vi "messageToCommand.vi"(7 "Self Enqueuer":refnum<class "Message Enqueuer.lvclass">, 8 "error in (no error)":errorcluster, 10 "Arguments":variant, 11 "Command":string) -> (0 "error out":errorcluster)   [LabVIEW 2017, in "BuildWorker.lvlib" / "BuildWorker.lvclass"]
uses:
  BuildWorker.lvclass
  <vilib>/ActorFramework/Message Enqueuer/Message Enqueuer.lvclass
  <vilib>/ActorFramework/Message Enqueuer/Message Enqueuer.lvclass/Message Enqueuer.ctl
  <vilib>/ActorFramework/Message Enqueuer/Enqueue.vi
  <vilib>/ActorFramework/Stop Msg/Stop Msg.lvclass
  Applications/National Instruments/LabVIEW 2017 64-bit/vi.lib/ActorFramework/Message/Message.lvclass
  WebSocket Server/Actors/Actor wHelper/Actor wUI Messages/Show UI Msg/Show UI Msg.lvclass
  <vilib>/ActorFramework/Message Priority Queue/Priority Enqueue.vi
  BuildWorker Messages/Name Request Msg/Name Request Msg.lvclass
  BuildWorker Messages/Remove Task Request Msg/Remove Task Request Msg.lvclass
  BuildWorker Messages/CurrentTaskName Request Msg/CurrentTaskName Request Msg.lvclass
  BuildWorker Messages/New Task Request Msg/New Task Request Msg.lvclass
  BuildWorker Messages/Enqueue Task List Msg/Enqueue Task List Msg.lvclass
  BuildWorker Messages/Abort Msg/Abort Msg.lvclass
  BuildWorker Messages/Send Worker Status Update Msg/Send Worker Status Update Msg.lvclass
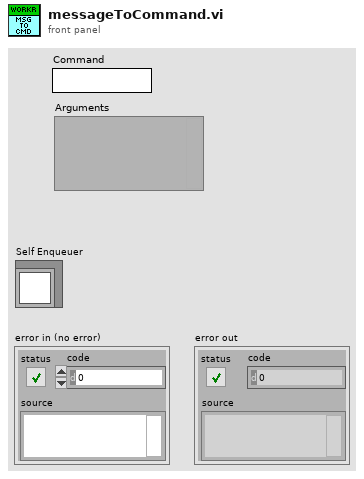
[diagram p1: front panel]
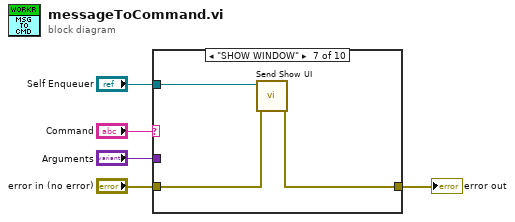
[diagram p0: block diagram]
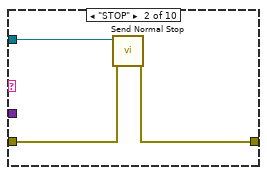
[diagram p3: hidden frame]
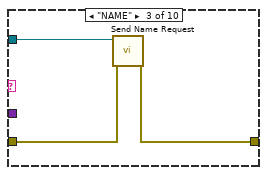
[diagram p4: hidden frame]
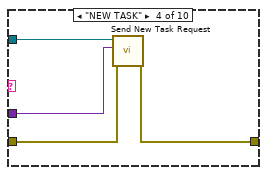
[diagram p5: hidden frame]
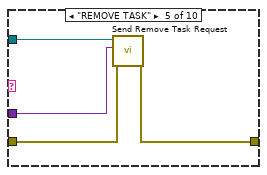
[diagram p6: hidden frame]
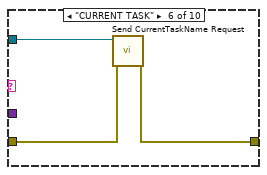
[diagram p7: hidden frame]
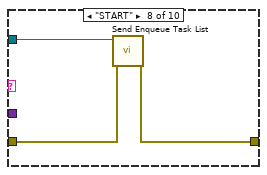
[diagram p8: hidden frame]
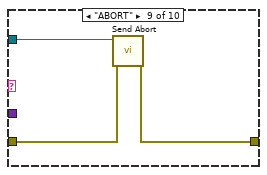
[diagram p9: hidden frame]
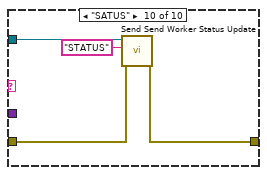
[diagram p10: hidden frame]
diagram:
  n1 = case shown="\"SHOW WINDOW\"" "Command" {
    tunnel: "Self Enqueuer" -> [_ w9 w12 w16 w20 w23 w26 w29 w32 w36]
    tunnel: "error in (no error)" -> [w6 w8 w11 w15 w19 w22 w25 w28 w31 w35]
    tunnel: [w6 w7 w10 w14 w18 w21 w24 w27 w30 w34] -> w3
    tunnel: "Arguments" -> [_ _ _ w13 w17 _ _ _ _ _]
    frame Default {
    }
    frame "STOP" {
      n2 = call <vilib>:"Send Normal Stop.vi"("error in (no error)"=w8, "Message Enqueuer"=w9) -> ("error out"=w7:errorcluster)  [unwired: 9 in]
    }
    frame "NAME" {
      n3 = call "Send Name Request.vi"("error in (no error)"=w11, "Message Enqueuer in"=w12) -> ("error out"=w10:errorcluster)  [unwired: 8 in, 1 out]
    }
    frame "NEW TASK" {
      n4 = call "Send New Task Request.vi"("error in (no error)"=w15, "Task"=w13, "Message Enqueuer in"=w16) -> ("error out"=w14:errorcluster)  [unwired: 7 in, 1 out]
    }
    frame "REMOVE TASK" {
      n5 = call "Send Remove Task Request.vi"("error in (no error)"=w19, "Task"=w17, "Message Enqueuer in"=w20) -> ("error out"=w18:errorcluster)  [unwired: 7 in, 1 out]
    }
    frame "CURRENT TASK" {
      n6 = call "Send CurrentTaskName Request.vi"("error in (no error)"=w22, "Message Enqueuer in"=w23) -> ("error out"=w21:errorcluster)  [unwired: 8 in, 1 out]
    }
    frame "SHOW WINDOW" {
      n7 = call "Send Show UI.vi"("error in (no error)"=w25, "Message Enqueuer"=w26) -> ("error out"=w24:errorcluster)  [unwired: 8 in, 1 out]
    }
    frame "START" {
      n8 = call "Send Enqueue Task List.vi"("error in (no error)"=w28, "Message Enqueuer in"=w29) -> ("error out"=w27:errorcluster)  [unwired: 8 in, 1 out]
    }
    frame "ABORT" {
      n9 = call "Send Abort.vi"("error in (no error)"=w31, "Message Enqueuer in"=w32) -> ("error out"=w30:errorcluster)  [unwired: 8 in, 1 out]
    }
    frame "SATUS" {
      n10 = call "Send Send Worker Status Update.vi"("error in (no error)"=w35, "Operation"="STATUS", "Message Enqueuer in"=w36) -> ("error out"=w34:errorcluster)  [unwired: 7 in, 1 out]
    }
  }
  "error out" <- w3
